vi "Export Trigger from Load for DMM Synchronization.vi"(8 "error in (no error)":errorcluster, 10 "DMM Trigger Source":T1(ring), 11 "Reference values":T2={"dcpower session reservation"=refnum, "Source handle array"=[], "Source channel name array"=[], "Load handle"="", "Load channel name"="", "Source voltage values"=[], "Load current values"=[], "Number of steps"=0, "Source sequence name"="", "Source terminal name"="", "Measure terminal name"="", "scope session reservation"=refnum, "Scope handles"=[], "connection map"={}, "instrument info map array"=[], "Enable TClk"=FALSE, "dmm session reservation"=refnum, "dmm handle array"=[], "DMM Trigger Source"=enum."Immediate", "DMM Sample Trigger"=enum."TTL 0", "Measurement Results"={"Status"="", "Voltage values"=[], "Source sweep points"=0, "Load sweep points"=0, "Source voltages"=[], "Source currents"=[], "Load voltages"=[], "Load currents"=[], "Load voltage deviation"=[], "Efficiency"=[], "Maximum efficiency"=[], "Minimum load voltage"=[], "Maximum load voltage"=[], "Minimum load regulation"=[], "Maximum load regulation"=[], "waveform pins"=[], "waveform sites"=[], "waveform t0 array"=[], "waveform dt array"=[], "waveform length array"=[], "concatenated waveform Y"=[]}, "Additional measurements"={"voltage measurements from all sources"=[], "current measurements from all sources"=[], "all dmm measurements"=[], "all scope waverforms"=[]}}) -> (0 "error out":errorcluster, 3 "Reference values out":T2={"dcpower session reservation"=refnum, "Source handle array"=[], "Source channel name array"=[], "Load handle"="", "Load channel name"="", "Source voltage values"=[], "Load current values"=[], "Number of steps"=0, "Source sequence name"="", "Source terminal name"="", "Measure terminal name"="", "scope session reservation"=refnum, "Scope handles"=[], "connection map"={}, "instrument info map array"=[], "Enable TClk"=FALSE, "dmm session reservation"=refnum, "dmm handle array"=[], "DMM Trigger Source"=enum."Immediate", "DMM Sample Trigger"=enum."TTL 0", "Measurement Results"={"Status"="", "Voltage values"=[], "Source sweep points"=0, "Load sweep points"=0, "Source voltages"=[], "Source currents"=[], "Load voltages"=[], "Load currents"=[], "Load voltage deviation"=[], "Efficiency"=[], "Maximum efficiency"=[], "Minimum load voltage"=[], "Maximum load voltage"=[], "Minimum load regulation"=[], "Maximum load regulation"=[], "waveform pins"=[], "waveform sites"=[], "waveform t0 array"=[], "waveform dt array"=[], "waveform length array"=[], "concatenated waveform Y"=[]}, "Additional measurements"={"voltage measurements from all sources"=[], "current measurements from all sources"=[], "all dmm measurements"=[], "all scope waverforms"=[]}})   [LabVIEW 2021, in "Efficiency And Load Regulation with Pin Map.lvlib"]
uses:
  Efficiency And Load Regulation with Pin Map.lvlib
  Reference values.ctl
  <vilib>/Plug-In SDKs/Clients/Session Management V1/Session Reservation/Session Reservation.lvclass
  common/Instrument Control/Scope/TClk/Instrument Info.ctl
  common/Instrument Control/Scope Parameters.ctl
  <instrlib>/niScope/Controls/niScope vertical coupling.ctl
  <instrlib>/niDMM/nidmm.llb/niDMM Sample Trigger.ctl
  Measurement Results.ctl
  Additional measurements.ctl
  <instrlib>/niDCPower/nidcpower.llb/niDCPower Export Signal - Signal.ctl
  <instrlib>/niDMM/nidmm.llb/niDMM Trigger.ctl
  common/PMIC Common.lvlib
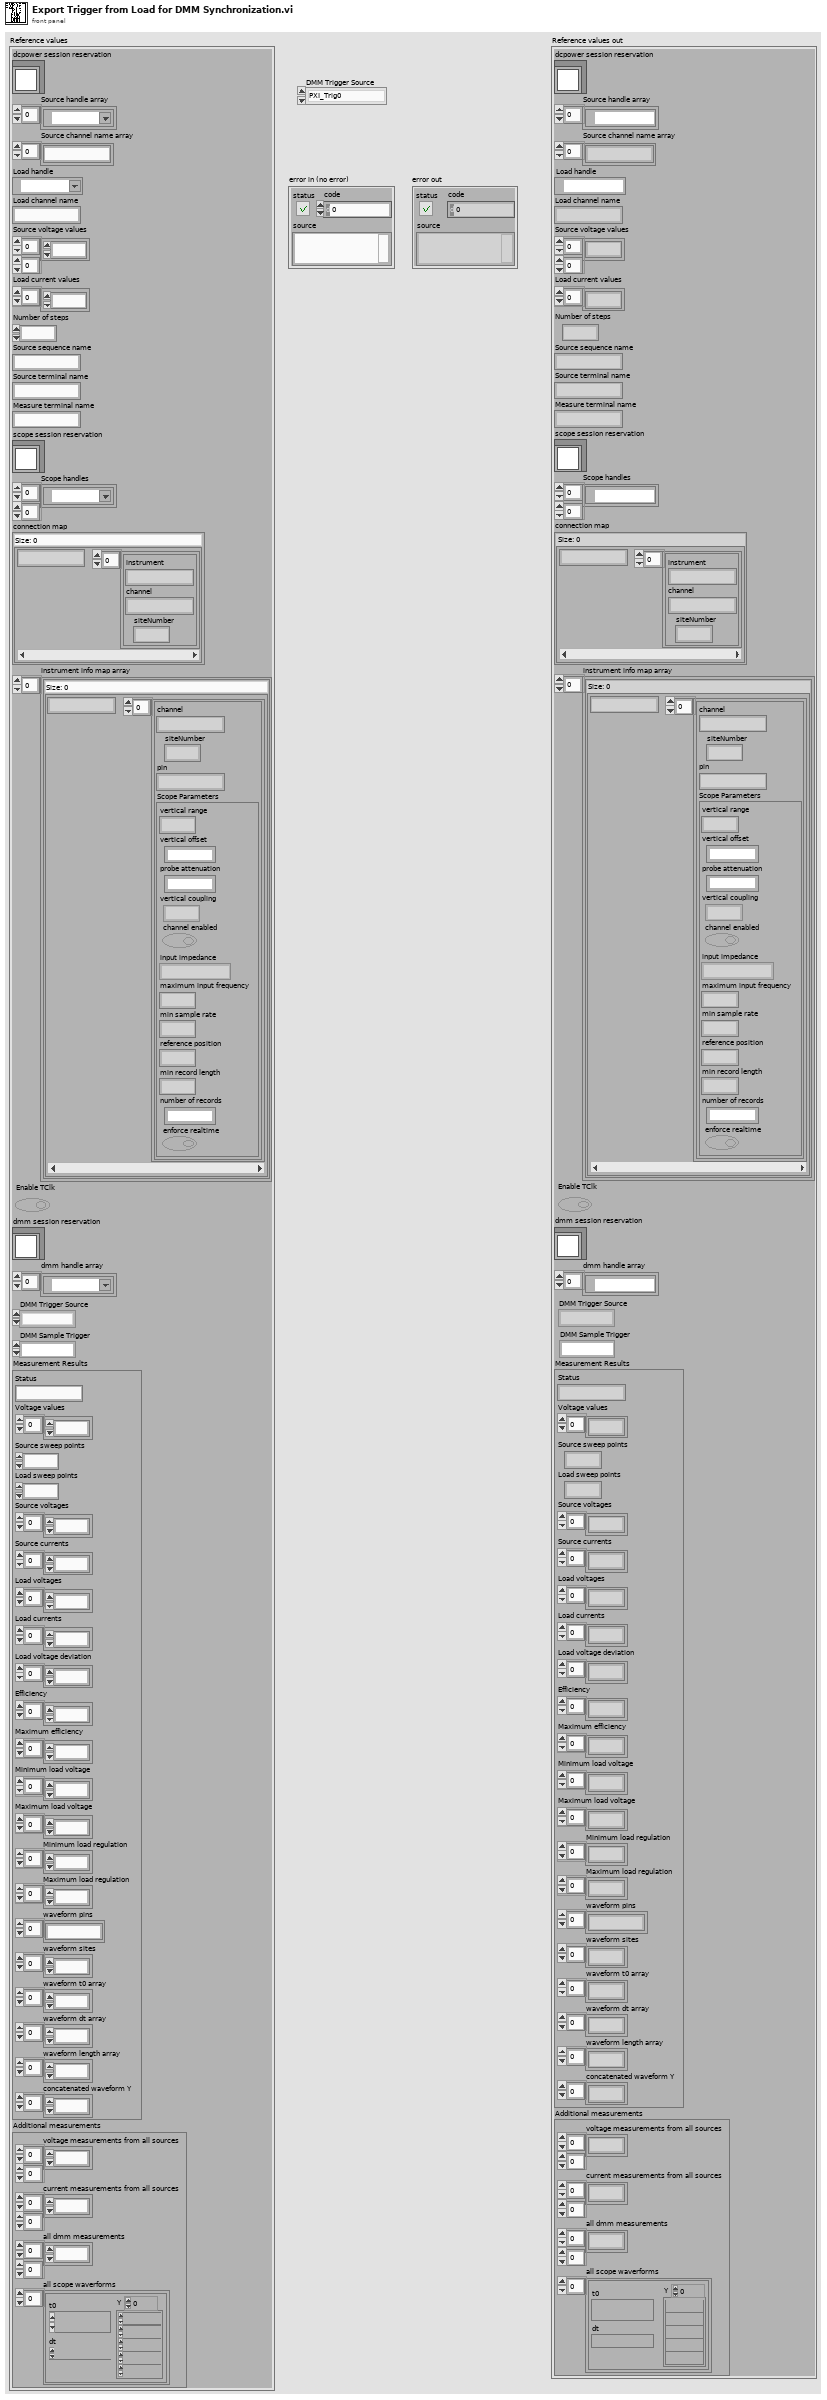
[diagram p1: front panel]
types:
  T1 = enum16{"PXI_Trig0", "PXI_Trig1", "PXI_Trig2", "PXI_Trig3", "PXI_Trig4", "PXI_Trig5", "PXI_Trig6", "PXI_Trig7"}
  T2 = typedef "Efficiency And Load Regulation with Pin Map.lvlib/Reference values.ctl" = cluster{"dcpower session reservation":refnum<class "Session Reservation.lvclass">, "Source handle array":refnum<k15>[], "Source channel name array":string[], "Load handle":refnum<k15>, "Load channel name":string, "Source voltage values":dbl[][], "Load current values":dbl[], "Number of steps":i32, "Source sequence name":string, "Source terminal name":string, "Measure terminal name":string, "scope session reservation":refnum<class "Session Reservation.lvclass">, "Scope handles":refnum<k15>[][], "connection map":map{string, T3[]}, "instrument info map array":map{string, cluster{"channel":string, "siteNumber":i32, "pin":string, "Scope Parameters":T4}[]}[], "Enable TClk":bool, "dmm session reservation":refnum<class "Session Reservation.lvclass">, "dmm handle array":refnum<k15>[], "DMM Trigger Source":T6, "DMM Sample Trigger":T7, "Measurement Results":T8, "Additional measurements":T9}
  T3 = typedef "PMIC Common.lvlib/Instrument Info.ctl" = cluster{"instrument":string, "channel":string, "siteNumber":i32}
  T4 = typedef "PMIC Common.lvlib/Scope Parameters.ctl" = cluster{"vertical range":dbl, "vertical offset":dbl, "probe attenuation":dbl, "vertical coupling":T5, "channel enabled":bool, "input impedance":u32, "maximum input frequency":dbl, "min sample rate":dbl, "reference position":dbl, "min record length":i32, "number of records":i32, "enforce realtime":bool}
  T5 = typedef "niScope vertical coupling.ctl" = i32
  T6 = typedef "niDMM Trigger.ctl" = enum16{"Immediate", "External", "TTL 0", "TTL 1", "TTL 2", "TTL 3", "TTL 4", "TTL 5", "TTL 6", "Software", "TTL 7", "PXI Star", "LBR Trig 1", "Aux Trig 1"}
  T7 = typedef "niDMM Sample Trigger.ctl" = enum16{"Immediate", "External", "TTL 0", "TTL 1", "TTL 2", "TTL 3", "TTL 4", "TTL 5", "TTL 6", "Interval", "Software", "TTL 7", "PXI Star", "LBR Trig 1", "Aux Trig 1"}
  T8 = typedef "Efficiency And Load Regulation with Pin Map.lvlib/Measurement Results.ctl" = cluster{"Status":string, "Voltage values":dbl[], "Source sweep points":i32, "Load sweep points":i32, "Source voltages":dbl[], "Source currents":dbl[], "Load voltages":dbl[], "Load currents":dbl[], "Load voltage deviation":dbl[], "Efficiency":dbl[], "Maximum efficiency":dbl[], "Minimum load voltage":dbl[], "Maximum load voltage":dbl[], "Minimum load regulation":dbl[], "Maximum load regulation":dbl[], "waveform pins":string[], "waveform sites":i32[], "waveform t0 array":dbl[], "waveform dt array":dbl[], "waveform length array":i32[], "concatenated waveform Y":dbl[]}
  T9 = typedef "Efficiency And Load Regulation with Pin Map.lvlib/Additional measurements.ctl" = cluster{"voltage measurements from all sources":dbl[][], "current measurements from all sources":dbl[][], "all dmm measurements":dbl[][], "all scope waverforms":waveform(dbl)[]}
  T10 = typedef "niDCPower Export Signal - Signal.ctl" = i32
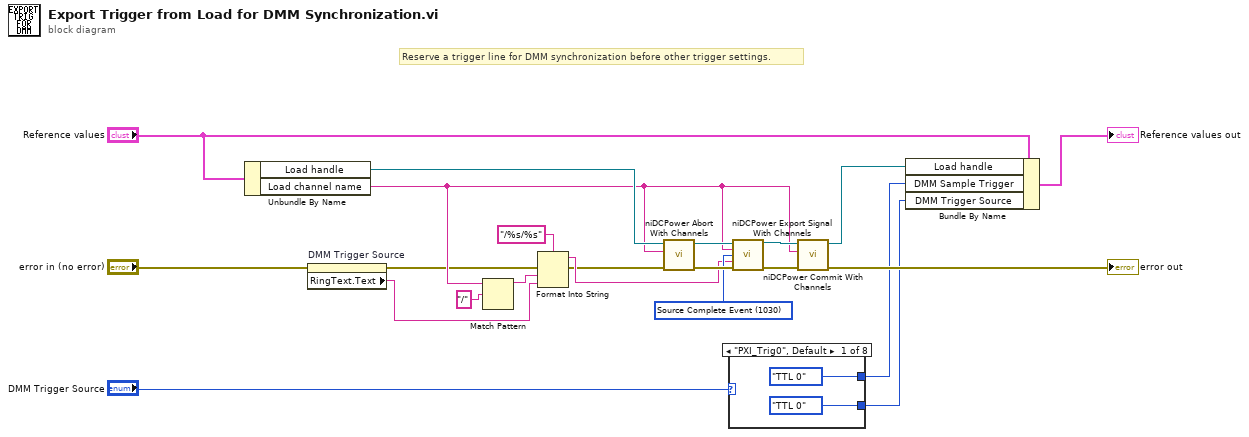
[diagram p0: block diagram]
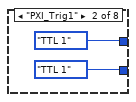
[diagram p2: hidden frame]
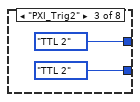
[diagram p3: hidden frame]
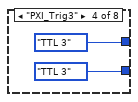
[diagram p4: hidden frame]
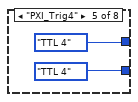
[diagram p5: hidden frame]
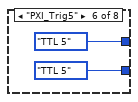
[diagram p6: hidden frame]
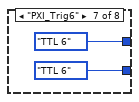
[diagram p7: hidden frame]
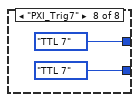
[diagram p8: hidden frame]
diagram:
  w16 = T10 1030 items=["Source Complete Event"=1030, "Measure Complete Event"=1031, "Sequence Iteration Complete Event"=1032, "Sequence Engine Done Event"=1033, "Pulse Complete Event"=1051, "Ready For Pulse Trigger Event"=1052, "Start Trigger"=1034, "Source Trigger"=1035, "Measure Trigger"=1036, "Sequence Advance Trigger"=1037, "Pulse Trigger"=1053] ("signal")
  # "Reserve a trigger line for DMM synchronization before other trigger settings."
  n1 = Unbundle By Name("Reference values") -> ("Load handle"=w13:refnum<k15>, "Load channel name"=w8:string)
  n2 = property on="DMM Trigger Source" class="Enum (strict)"(error in="error in (no error)") -> (error out=w5:errorcluster, "RingText.Text"=w4:string)  [unwired: 1 in, 1 out]
  n3 = Match Pattern(string=w8, regular expression="/") -> (before substring=w11:string)  [unwired: 1 in, 3 out]
  n4 = Format Into String(format string="/%s/%s", error in=w5, w11, w4) -> (resulting string=w7:string, error out=w6:errorcluster)  [unwired: 1 in]
  n5 = call <instrlib>:"niDCPower Abort With Channels.vi"("error in (no error)"=w6, "channel name"=w8, "instrument handle"=w13) -> ("error out"=w18:errorcluster, "instrument handle out"=w17:refnum<k15>)  [unwired: 7 in]
  n6 = case shown="\"PXI_Trig0\", Default" "DMM Trigger Source" {
    tunnel: [niDMM_Sample_Trigger."TTL 0" ("DMM Sample Trigger") niDMM_Sample_Trigger."TTL 1" ("DMM Sample Trigger") niDMM_Sample_Trigger."TTL 2" ("DMM Sample Trigger") niDMM_Sample_Trigger."TTL 3" ("DMM Sample Trigger") niDMM_Sample_Trigger."TTL 4" ("DMM Sample Trigger") niDMM_Sample_Trigger."TTL 5" ("DMM Sample Trigger") niDMM_Sample_Trigger."TTL 6" ("DMM Sample Trigger") niDMM_Sample_Trigger."TTL 7" ("DMM Sample Trigger")] -> w2
    tunnel: [niDMM_Trigger."TTL 0" ("DMM Trigger Source") niDMM_Trigger."TTL 1" ("DMM Trigger Source") niDMM_Trigger."TTL 2" ("DMM Trigger Source") niDMM_Trigger."TTL 3" ("DMM Trigger Source") niDMM_Trigger."TTL 4" ("DMM Trigger Source") niDMM_Trigger."TTL 5" ("DMM Trigger Source") niDMM_Trigger."TTL 6" ("DMM Trigger Source") niDMM_Trigger."TTL 7" ("DMM Trigger Source")] -> w1
    frame "PXI_Trig0", Default {
    }
    frame "PXI_Trig1" {
    }
    frame "PXI_Trig2" {
    }
    frame "PXI_Trig3" {
    }
    frame "PXI_Trig4" {
    }
    frame "PXI_Trig5" {
    }
    frame "PXI_Trig6" {
    }
    frame "PXI_Trig7" {
    }
  }
  n7 = call <instrlib>:"niDCPower Export Signal With Channels.vi"("instrument handle"=w17, "channel name"=w8, "signal"=w16, "output terminal"=w7, "error in (no error)"=w18) -> ("instrument handle out"=w14:refnum<k15>, "error out"=w15:errorcluster)  [unwired: 9 in]
  n8 = call <instrlib>:"niDCPower Commit With Channels.vi"("error in (no error)"=w15, "channel name"=w8, "instrument handle"=w14) -> ("error out"=→"error out":errorcluster, "instrument handle out"=w12:refnum<k15>)  [unwired: 7 in]
  n9 = Bundle By Name(cluster="Reference values", "Load handle"=w12, "DMM Sample Trigger"=w2, "DMM Trigger Source"=w1) -> (→"Reference values out":T2)
